vi "Deconstruct.vi"(0 "Export In":refnum<class "Export.lvclass">) -> ()   [LabVIEW 2017, in "CL_G3_VIComponentBuilder.lvlib" / "Export.lvclass"]
doc: "Destroys the Export object."
uses:
  Export.lvclass
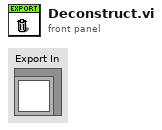
[diagram p1: front panel]
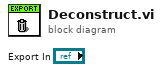
[diagram p0: block diagram]
diagram:
